vi "RealEncoderTest.vi"() -> ()   [LabVIEW 2010]
uses:
  <vilib>/eio/EIONode/EIONode.xnode
  <vilib>/rvi/eio/nirviEIOImplementation/nirviEIOImplementation.xnode
  <vilib>/rvi/eio/common/nirviEmuTemplateMethod_noerrors.vi
  <vilib>/rvi/eio/common/nirviEmuClasses.ctl
  Motor Control/Motor Global.vi
panel:
  out "Reset Steering due to index?":bool
  in  "Use Steering Index to reset":bool
  out "Reset Lidar due to index?":bool
  in  "Use Lidar Index to reset":bool
  in  "Use Drive Index to reset":bool
  out "Reset Drive due to index?":bool
  out "The Steering Encoder Changed":bool
  out "Current Steering Encoder Value":i32
  out "Maximum Steering Encoder Count":i32
  out "Minimum Steering Encoder Count":i32
  out "The Lidar Encoder Changed":bool
  out "Current Lidar Encoder Value":i32
  out "Maximum Lidar Encoder Count":i32
  out "Minimum Lidar Encoder Count":i32
  out "Minimum Drive Encoder Count":i32
  out "Maximum Drive Encoder Count":i32
  out "Current Drive Encoder Value":i32
  out "The Drive Encoder Changed":bool
  out "Steering Encoder A":bool
  out "Steering Encoder B":bool
  out "Steering Encoder Index":bool
  out "Lidar Encoder A":bool
  out "Lidar Encoder B":bool
  out "Lidar Encoder Index":bool
  out "Drive Encoder A":bool
  out "Drive Encoder B":bool
  out "Drive Encoder Index":bool
  in  "stop":bool
  in  "Lidar Enable":bool
  in  "Steering Enable":bool
  in  "Drive Enable":bool
  in  "Lidar output Voltage":fxp<+/-,20,5>
  in  "Steering output Voltage":fxp<+/-,20,5>
  in  "Drive output Voltage":fxp<+/-,20,5>
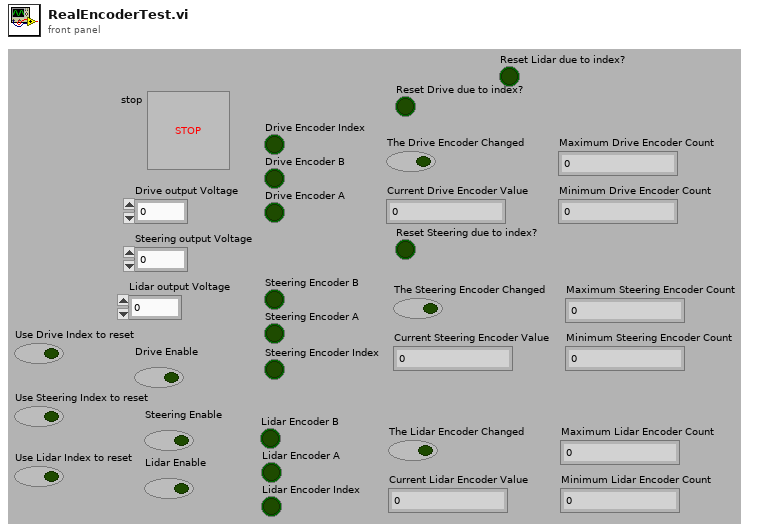
[diagram p1: front panel]
types:
  T1 = typedef "nirviEmuClasses.ctl" = enum16{"IO Read", "IO Write", "Method", "Property Read", "Property Write"}
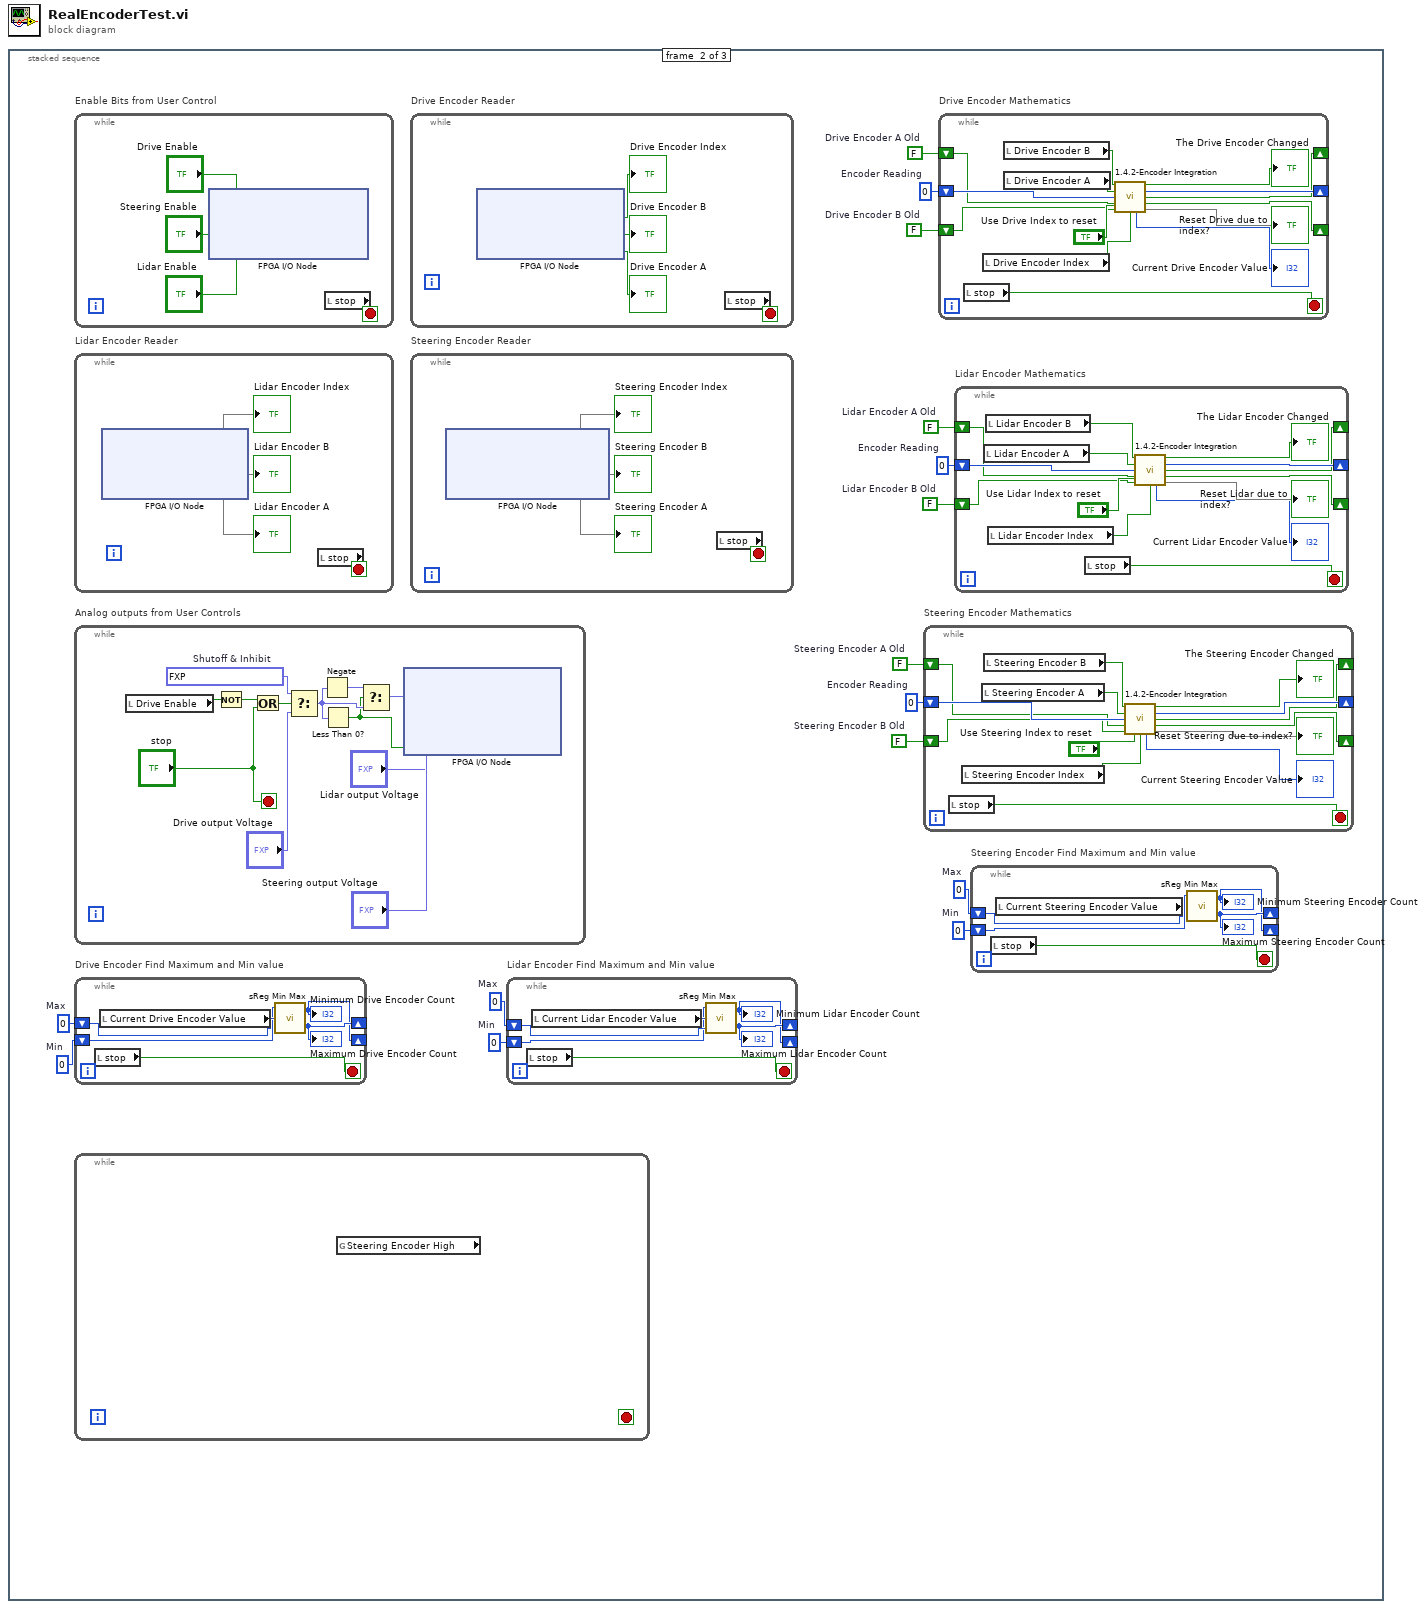
[diagram p0: block diagram]
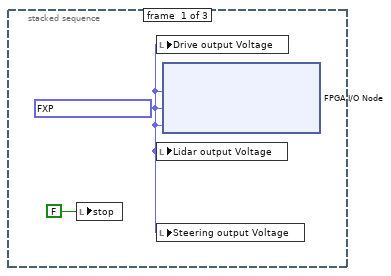
[diagram p2: hidden frame]
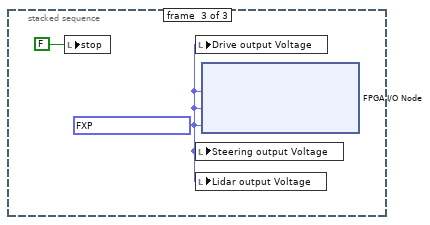
[diagram p3: hidden frame]
diagram:
  n1 = stacked-sequence {
    frame #0 {
      w1 = fxp<+/-,20,5> 0.0 ("Steering output Voltage")
      n2 = local write "stop"(FALSE ("stop")) -> ()
      n3 = local write "Drive output Voltage"(w1) -> ()
      n4 = local write "Lidar output Voltage"(w1) -> ()
      n5 = local write "Steering output Voltage"(w1) -> ()
      n6 = xnode "FPGA I/O Node"("Drive Motor Speed"=w1, "Steering Motor Speed"=w1, "Lidar Motor Speed"=w1) -> ()  [unwired: 3 in, 3 out]
    }
    frame #1 {
      w6 = 0  # Min
      w7 = 0  # Max
      w8 = 0  # Encoder Reading
      w9 = FALSE  # Steering Encoder A Old
      w10 = FALSE  # Steering Encoder B Old
      w15 = 0  # Min
      w14 = 0  # Max
      w13 = 0  # Encoder Reading
      w12 = FALSE  # Lidar Encoder A Old
      w11 = FALSE  # Lidar Encoder B Old
      w16 = 0  # Min
      w17 = 0  # Max
      w18 = 0  # Encoder Reading
      w19 = FALSE  # Drive Encoder A Old
      w20 = FALSE  # Drive Encoder B Old
      n7 = while "Enable Bits from User Control" {
        stop <- w172 stop-if-true
        n8 = xnode "FPGA I/O Node"("Drive Motor Enable"="Drive Enable", "Steering Motor Inhibit"="Steering Enable", "Lidar Motor Inhibit"="Lidar Enable") -> ()  [unwired: 3 in, 3 out]
        n9 = local read "stop"() -> (w172:bool)
      }
      n10 = while "Lidar Encoder Reader" {
        stop <- w91 stop-if-true
        n11 = xnode "FPGA I/O Node"() -> ("Lidar Encoder Index"=→"Lidar Encoder Index", "Lidar Encoder B"=→"Lidar Encoder B", "Lidar Encoder A"=→"Lidar Encoder A")  [unwired: 3 in, 3 out]
        n12 = local read "stop"() -> (w91:bool)
      }
      n13 = while "Analog outputs from User Controls" {
        stop <- "stop" stop-if-true
        w164 = fxp<+/-,20,5> 0.0  # Shutoff & Inhibit
        n14 = local read "Drive Enable"() -> (w162:bool)
        n15 = Not(x=w162) -> (.not. x?=w161:bool)
        n16 = Or(x=w161, y="stop") -> (x .or. y?=w160:bool)
        n17 = Select(t=w164, s=w160, f="Drive output Voltage") -> (s? t:f=w158:fxp<+/-,20,5>)
        n18 = Negate(x=w158) -> (-x=w157:fxp<+/-,20,5>)
        n19 = Less Than 0?(x=w158) -> (x < 0?=w156:bool)
        n20 = Select(t=w157, s=w156, f=w158) -> (s? t:f=w159:fxp<+/-,20,5>)
        n21 = xnode "FPGA I/O Node"("Drive Motor Speed"=w159, "Steering Motor Speed"="Steering output Voltage", "Lidar Motor Speed"="Lidar output Voltage", "Drive Motor Reverse"=w156) -> ()  [unwired: 4 in, 4 out]
      }
      n22 = while "Drive Encoder Find Maximum and Min value" {
        shift-right: [w62] -> _
        shift-left: w17 -> [w63]
        shift-right: [w61] -> _
        shift-left: w16 -> [w64]
        stop <- w66 stop-if-true
        n23 = local read "stop"() -> (w66:bool)
        n24 = local read "Current Drive Encoder Value"() -> (w65:i32)
        n25 = call "sReg Min Max.vi"("Max from sReg"=w63, "New Value"=w65, "Min from sReg"=w64) -> ("Max to sReg"=w62:i32, "Min to sReg"=w61:i32)
        "Maximum Drive Encoder Count" <- w62
        "Minimum Drive Encoder Count" <- w61
      }
      n26 = while {
        stop <- _ stop-if-true
        n27 = global read "Motor Global.vi" "Steering Encoder High"() -> ()  [unwired: 1 out]
      }
      n28 = while "Drive Encoder Reader" {
        stop <- w98 stop-if-true
        n29 = xnode "FPGA I/O Node"() -> ("Drive Encoder Index"=→"Drive Encoder Index":bool, "Drive Encoder B"=→"Drive Encoder B":bool, "Drive Encoder A"=→"Drive Encoder A":bool)  [unwired: 3 in, 3 out]
        n30 = local read "stop"() -> (w98:bool)
      }
      n31 = while "Steering Encoder Reader" {
        stop <- w84 stop-if-true
        n32 = xnode "FPGA I/O Node"() -> ("Steering Encoder Index"=→"Steering Encoder Index", "Steering Encoder B"=→"Steering Encoder B", "Steering Encoder A"=→"Steering Encoder A")  [unwired: 3 in, 3 out]
        n33 = local read "stop"() -> (w84:bool)
      }
      n34 = while "Lidar Encoder Find Maximum and Min value" {
        shift-right: [w45] -> _
        shift-left: w14 -> [w46]
        shift-right: [w42] -> _
        shift-left: w15 -> [w43]
        stop <- w41 stop-if-true
        n35 = local read "stop"() -> (w41:bool)
        n36 = local read "Current Lidar Encoder Value"() -> (w44:i32)
        n37 = call "sReg Min Max.vi"("Max from sReg"=w46, "New Value"=w44, "Min from sReg"=w43) -> ("Max to sReg"=w45:i32, "Min to sReg"=w42:i32)
        "Maximum Lidar Encoder Count" <- w45
        "Minimum Lidar Encoder Count" <- w42
      }
      n38 = while "Steering Encoder Mathematics" {
        shift-right: [w33] -> _
        shift-left: w9 -> [w28]
        shift-right: [w32] -> _
        shift-left: w10 -> [w27]
        shift-right: [w36] -> _
        shift-left: w8 -> [w37]
        stop <- w40 stop-if-true
        n39 = local read "stop"() -> (w40:bool)
        n40 = local read "Steering Encoder Index"() -> (w30:bool)
        n41 = local read "Steering Encoder A"() -> (w38:bool)
        n42 = local read "Steering Encoder B"() -> (w39:bool)
        n43 = call "1.4.2-Encoder Integration.vi"("Encoder B"=w39, "Encoder A"=w38, 7:w37, "Encoder A Old"=w28, "Encoder B Old"=w27, 12:"Use Steering Index to reset", "Encoder Index"=w30) -> ("The Encoder Changed"=→"The Steering Encoder Changed":bool, "Count Zeroed at Index"=w36:i32, "Encoder A Old (sReg)"=w33:bool, "Encoder B Old (sReg)"=w32:bool, "Current count"=→"Current Steering Encoder Value":i32, 15:→"Reset Steering due to index?")  [unwired: 2 in, 1 out]
      }
      n44 = while "Drive Encoder Mathematics" {
        shift-right: [w73] -> _
        shift-left: w19 -> [w71]
        shift-right: [w69] -> _
        shift-left: w20 -> [w67]
        shift-right: [w78] -> _
        shift-left: w18 -> [w80]
        stop <- w77 stop-if-true
        n45 = local read "stop"() -> (w77:bool)
        n46 = local read "Drive Encoder Index"() -> (w75:bool)
        n47 = local read "Drive Encoder B"() -> (w68:bool)
        n48 = local read "Drive Encoder A"() -> (w72:bool)
        n49 = call "1.4.2-Encoder Integration.vi"("Encoder B"=w68, "Encoder A"=w72, 7:w80, "Encoder A Old"=w71, "Encoder B Old"=w67, 12:"Use Drive Index to reset", "Encoder Index"=w75) -> ("The Encoder Changed"=→"The Drive Encoder Changed":bool, "Count Zeroed at Index"=w78:i32, "Encoder A Old (sReg)"=w73:bool, "Encoder B Old (sReg)"=w69:bool, "Current count"=→"Current Drive Encoder Value":i32, 15:→"Reset Drive due to index?")  [unwired: 2 in, 1 out]
      }
      n50 = while "Lidar Encoder Mathematics" {
        shift-right: [w54] -> _
        shift-left: w12 -> [w48]
        shift-right: [w53] -> _
        shift-left: w11 -> [w47]
        shift-right: [w56] -> _
        shift-left: w13 -> [w57]
        stop <- w60 stop-if-true
        n51 = local read "Lidar Encoder A"() -> (w58:bool)
        n52 = local read "Lidar Encoder B"() -> (w59:bool)
        n53 = local read "Lidar Encoder Index"() -> (w50:bool)
        n54 = local read "stop"() -> (w60:bool)
        n55 = call "1.4.2-Encoder Integration.vi"("Encoder B"=w59, "Encoder A"=w58, 7:w57, "Encoder A Old"=w48, "Encoder B Old"=w47, 12:"Use Lidar Index to reset", "Encoder Index"=w50) -> ("The Encoder Changed"=→"The Lidar Encoder Changed":bool, "Count Zeroed at Index"=w56:i32, "Encoder A Old (sReg)"=w54:bool, "Encoder B Old (sReg)"=w53:bool, "Current count"=→"Current Lidar Encoder Value":i32, 15:→"Reset Lidar due to index?")  [unwired: 2 in, 1 out]
      }
      n56 = while "Steering Encoder Find Maximum and Min value" {
        shift-right: [w22] -> _
        shift-left: w7 -> [w24]
        shift-right: [w21] -> _
        shift-left: w6 -> [w25]
        stop <- w26 stop-if-true
        n57 = local read "stop"() -> (w26:bool)
        n58 = local read "Current Steering Encoder Value"() -> (w23:i32)
        n59 = call "sReg Min Max.vi"("Max from sReg"=w24, "New Value"=w23, "Min from sReg"=w25) -> ("Max to sReg"=w22:i32, "Min to sReg"=w21:i32)
        "Maximum Steering Encoder Count" <- w22
        "Minimum Steering Encoder Count" <- w21
      }
    }
    frame #2 {
      w179 = fxp<+/-,20,5> 0.0 ("Lidar output Voltage")
      n60 = local write "stop"(FALSE ("stop")) -> ()
      n61 = local write "Drive output Voltage"(w179) -> ()
      n62 = local write "Steering output Voltage"(w179) -> ()
      n63 = local write "Lidar output Voltage"(w179) -> ()
      n64 = xnode "FPGA I/O Node"("Drive Motor Speed"=w179, "Steering Motor Speed"=w179, "Lidar Motor Speed"=w179) -> ()  [unwired: 3 in, 3 out]
    }
  }
